vi "Deallocate.vi"(8 "error in (no error)":errorcluster, 11 "Pointer in":refnum<class "Pointer.lvclass">) -> (0 "error out":errorcluster, 3 "Pointer out":refnum<class "Pointer.lvclass">)   [LabVIEW 2017, in "Memory Manager.lvlib" / "Pointer.lvclass"]
uses:
  Pointer.lvclass
  Protected/Error VIs/Zone.vi
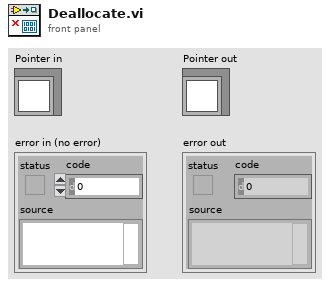
[diagram p1: front panel]
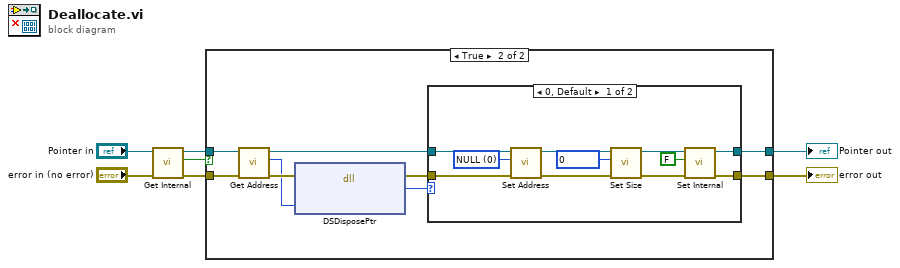
[diagram p0: block diagram]
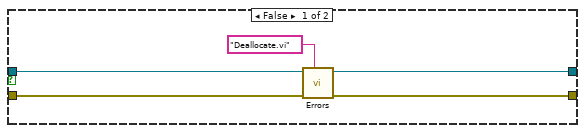
[diagram p2: hidden frame]
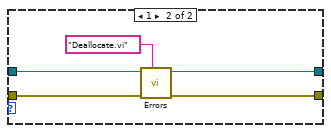
[diagram p3: hidden frame]
diagram:
  n1 = call "Get Internal.vi"("Pointer in"="Pointer in") -> ("internal"=w1:bool, "Pointer out"=w2:refnum<class "Pointer.lvclass">)  [unwired: 9 in]
  n2 = case shown="True" w1 {
    tunnel: [w8 w19] -> w6
    tunnel: [w7 w18] -> w5
    tunnel: "error in (no error)" -> [w9 w17]
    tunnel: w2 -> [w10 w12]
    frame False {
      n3 = call-poly "Errors.vi"("error source vi name"="Deallocate.vi" ("source vi name"), "error in (no error)"=w9, "Pointer in"=w10) -> ("error out"=w7:errorcluster, "Pointer out"=w8:refnum<class "Pointer.lvclass">)  [unwired: 7 in]
    }
    frame True {
      n4 = call "Get Address.vi"("Pointer in"=w12) -> ("address"=w13:u64, "Pointer out"=w14:refnum<class "Pointer.lvclass">)  [unwired: 9 in]
      n5 = dll-call lib="LabVIEW" fn="DSDisposePtr"(error in=w17, "pointer"=w13) -> (error out=w16:errorcluster, "return"=w15:i32)  [unwired: 3 in, 1 out]
      n6 = case shown="0, Default" w15 {
        tunnel: w16 -> [w23 w32]
        tunnel: [w23 w31] -> w18
        tunnel: [w21 w30] -> w19
        tunnel: w14 -> [w27 w29]
        frame 0, Default {
          w24 = u64 0 items=["NULL"] ("Null")
          n7 = call "Set Address.vi"("address"=w24, "Pointer in"=w27) -> ("Pointer out"=w26:refnum<class "Pointer.lvclass">)  [unwired: 9 in]
          n8 = call "Set Size.vi"("size"=u64 0, "Pointer in"=w26) -> ("Pointer out"=w22:refnum<class "Pointer.lvclass">)  [unwired: 9 in]
          n9 = call "Set Internal.vi"("internal"=FALSE, "Pointer in"=w22) -> ("Pointer out"=w21:refnum<class "Pointer.lvclass">)  [unwired: 9 in]
        }
        frame 1 {
          n10 = call-poly "Errors.vi"("error source vi name"="Deallocate.vi" ("source vi name"), "error in (no error)"=w32, "Pointer in"=w29) -> ("error out"=w31:errorcluster, "Pointer out"=w30:refnum<class "Pointer.lvclass">)  [unwired: 7 in]
        }
      }
    }
  }
  "error out" <- w5
  "Pointer out" <- w6
